vi "Trumpf_RD_DataBaseUpload.vi"(2 "error in (no error)":errorcluster, 3 "Bar_LIV_Data":path=path "D:/LabVIEW_prog/Trumpf_Database_Connect/TestData/Averaging_DM17-20_Post.xlsx") -> (0 "error out":errorcluster, 1 "Datasets Num":i32)   [LabVIEW 2017]
doc: "This example allows you to perform several tasks on the specified table in a database named LabVIEW.mdb located in the LabVIEW examples>>database directory.\n\nThis VI is running when you open it. Select one of the tabs and enter the appropriate data. Press the Go button to complete the displayed tab option.\n\nAutomatic - This option inserts a new record into the specified table. The record is specified by a cluster containing the correct number of elements and of the data types defined by the specified table. \n\nSQL Query - This option performs the specified SQL query.\n\nParameterized SQL Query - This option performs the specified SQL query as a parameterized SQL Query. This method is faster and more efficient than directly executing an SQL query because it sets up all the parameters prior to doing the command."
uses:
  <vilib>/addons/database/Connection.llb/DB Tools Open Connec (String).vi
  <vilib>/addons/database/NI_Database_API.lvlib
panel:
  out "Current value size":i32
  out "Database Column":string[](array[string])
  # "Overview: Demonstrates how to insert records into databases, and perform SQL queries.\nRequirements: Database Connectivity Toolkit\nInstructions:\nRun the VI."
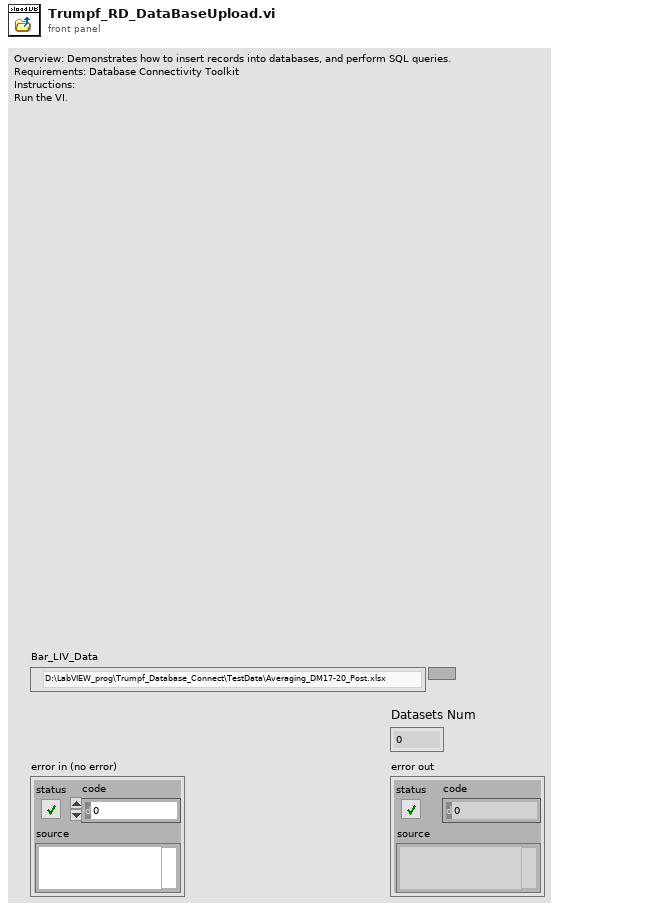
[diagram p1: front panel]
types:
  T1 = cluster{"Test Date":string, "Bar SN":string[], "Bar WO":string[], "Wafer ID":string[], "Last update":string[], "Current value(A)":dbl[], "Power(W)":dbl[][], "Voltage(V)":dbl[][], "Centroid(nm)":dbl[][], "Junction Temp(C)":dbl[][], "Efficiency(%)":dbl[][]}
  T2 = typedef "NI_Database_API.lvlib/Conn ObjectReference.ctl" = refnum<k1>
  T3 = cluster{"Test Date":string, string, string, string, string, dbl, dbl, dbl, dbl, dbl, dbl}
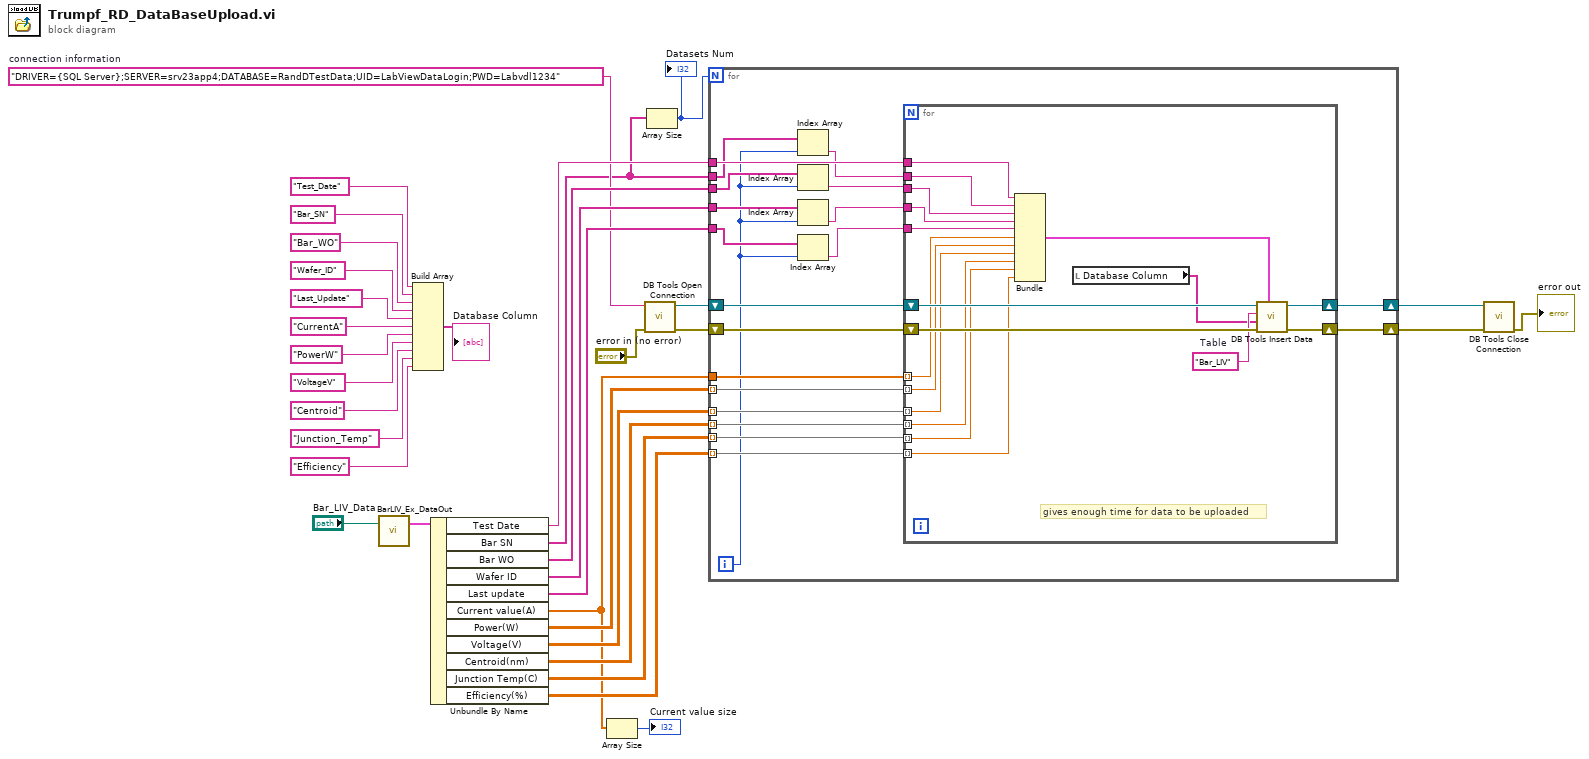
[diagram p0: block diagram]
diagram:
  w7 = "DRIVER={SQL Server};SERVER=srv23app4;DATABASE=RandDTestData;UID=LabViewDataLogin;PWD=Labvdl1234"  # connection information
  n1 = call "BarLIV_Ex_DataOut.vi"("Bar_LIV_Data"="Bar_LIV_Data") -> ("Output test data"=w29:T1)  [unwired: 1 in, 1 out]
  n2 = Build Array("Test_Date", "Bar_SN", "Bar_WO", "Wafer_ID", "Last_Update", "CurrentA", "PowerW", "VoltageV", "Centroid", "Junction_Temp", "Efficiency") -> (→"Database Column":string[])
  n3 = Unbundle By Name(w29) -> ("Test Date"=w28:string, "Bar SN"=w2:string[], "Bar WO"=w26:string[], "Wafer ID"=w25:string[], "Last update"=w24:string[], "Current value(A)"=w6:dbl[], "Power(W)"=w27:dbl[][], "Voltage(V)"=w23:dbl[][], "Centroid(nm)"=w22:dbl[][], "Junction Temp(C)"=w21:dbl[][], "Efficiency(%)"=w20:dbl[][])
  n4 = Array Size(array=w6) -> (size(s)=→"Current value size":i32)
  n5 = call-poly <vilib>:"DB Tools Open Connection.vi"("error in (no error)"="error in (no error)", "connection information"=w7) -> ("error out"=w31:errorcluster, "connection reference"=w32:T2)  [unwired: 6 in]
  n6 = Array Size(array=w2) -> (size(s)=w1:i32)
  "Datasets Num" <- w1
  n7 = for {
    N: w1 -> [_]
    shift-right: [w52] -> w33
    shift-left: w32 -> [w54]
    shift-right: [w51] -> w34
    shift-left: w31 -> [w53]
    tunnel: w28 -> [w50]
    tunnel: w6 -> [w49]
    tunnel: w27 -> [w48] mode=indexing
    tunnel: w2 -> [w43]
    tunnel: w26 -> [w42]
    tunnel: w25 -> [w41]
    tunnel: w24 -> [w40]
    tunnel: w23 -> [w47] mode=indexing
    tunnel: w22 -> [w46] mode=indexing
    tunnel: w21 -> [w45] mode=indexing
    tunnel: w20 -> [w44] mode=indexing
    i -> [w35]
    n8 = Index Array(array=w43, index=w35) -> (element=w39:string)
    n9 = Index Array(array=w42, index=w35) -> (element=w38:string)
    n10 = Index Array(array=w41, index=w35) -> (element=w37:string)
    n11 = Index Array(array=w40, index=w35) -> (element=w36:string)
    n12 = for {
      shift-right: [w69] -> w52
      shift-left: w54 -> [w72]
      shift-right: [w68] -> w51
      shift-left: w53 -> [w71]
      tunnel: w50 -> [w67]
      tunnel: w49 -> [w62] mode=indexing
      tunnel: w48 -> [w61] mode=indexing
      tunnel: w39 -> [w66]
      tunnel: w38 -> [w65]
      tunnel: w37 -> [w64]
      tunnel: w36 -> [w63]
      tunnel: w47 -> [w60] mode=indexing
      tunnel: w46 -> [w59] mode=indexing
      tunnel: w45 -> [w58] mode=indexing
      tunnel: w44 -> [w57] mode=indexing
      w70 = "Bar_LIV"  # Table
      # "gives enough time for data to be uploaded"
      n13 = Bundle("Test Date"=w67, w66, w65, w64, w63, w62, w61, w60, w59, w58, w57) -> (w56:T3)  [unwired: 1 in]
      n14 = local read "Database Column"() -> (w55:string[])
      n15 = call <vilib>:"DB Tools Insert Data.vi"("data"=w56, "error in (no error)"=w71, "columns"=w55, "table"=w70, "connection reference"=w72) -> ("error out"=w68:errorcluster, "connection reference out"=w69:T2)  [unwired: 5 in]
    }
  }
  n16 = call <vilib>:"DB Tools Close Connection.vi"("error in (no error)"=w34, "connection reference"=w33) -> ("error out"=→"error out":errorcluster)  [unwired: 5 in]
